vi "Initial_Plugin_Dynamixel.vi"() -> (5 "Plug in titles":string[](array[string]), 7 "Plug in values":string[](array[string]))   [LabVIEW 2022 SP3]
uses:
  Controls/Post_Process.ctl
  Controls/Setup.ctl
  Globals/Trav_pos_global.vi
  Globals/Meas_global.vi
  ADAM Serial/Instrument drivers/Dynamixel/Sub Vis/Dynamixel Global.vi
  <vilib>/ptbypt/NI_PtbyPt.lvlib
panel:
  out "On This Block":i32
  out "Amplitude":dbl
  out "Centre":dbl
  in  "Phase (Deg)":dbl
  in  "No of Cycles":dbl
  in  "Acceleration":dbl
  in  "Velocity":dbl
  in  "Min Peak":dbl
  in  "Max peak":dbl
  in  "Sinewave Freq (Hz)":dbl
  in  "Delay between Rendezvous and Acquisition starting (ms)":u32
  in  "Delay before each Traverse Move (ms)":u32=2000
  out "Position (Deg)":dbl
  out "Message":string
  out "Case Currently On":string
  # "The Vi\nEnFlo Software\\ADAM Serial\\Instrument drivers\\Dynamixel\\Dynamixel live Position Server.vi\nmust be running for this vi to work"
  # "Specific Arguments"
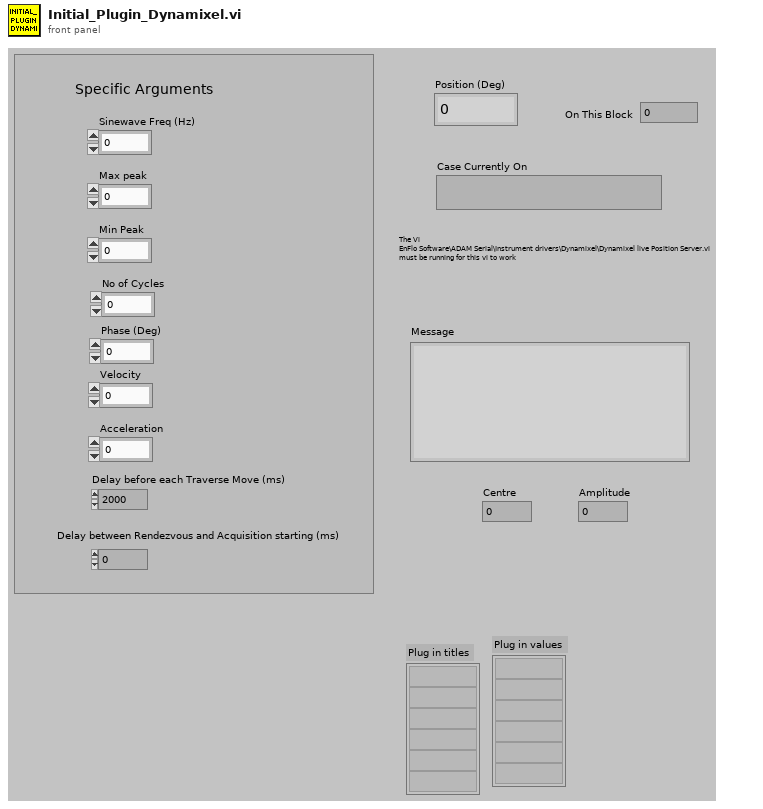
[diagram p1: front panel]
types:
  T1 = typedef "Traverse_cluster.ctl" = cluster{"Start X":sgl, "Start Y":sgl, "Start Z":sgl, "End X":sgl, "End Y":sgl, "End Z":sgl, "nPoints":i32, "Spacing":T2, "Filename":path, "Tunnel Speed":dbl, "Averaging time (mins)":dbl, "Extra Commands":string, "Carrier_1 Q (l/min)":dbl, "Carrier_2 Q (l/min)":dbl, "Trace Gas Concentration (%)":dbl, "Specific Arguments":string, "Comments":string, "Row No":i32, "Row Type Selector":T3, "EstCompl":string, "Row Duration (mins)":dbl, "nValidPoints":i32, "Meas Setup File":string}
  T2 = typedef "Spacing.ctl" = enum16{"Linear", "Log", "Gauss", "Specified", "N/A"}
  T3 = typedef "Multi_run_mode.ctl" = enum16{"Move Traverse Only", "Set Tunnel Speed Only", "Set Source Only", "Set Measurement Conditions", "Single Measurement", "Vertical Profile", "Lateral Profile", "Longitudinal Profile", "Multi-Axis Profile", "Explore Volume", "Auto Calibrate", "Meas Fast FID Bkgnd", "Check Beam Power", "Scanning Valve Measurement", "Run VI Named:", "Set ADAM Ch", "Wait (minutes)", "Send Message", "Synchronize With:", "Fall Back to this Row", "Turn Off Row Repeating", "Traverse 3D Volume", "Blank Row", "Jump to Fall Back Row"}
  T4 = typedef "Post_Process.ctl" = enum16{"Take New Data", "Post Process Raw Data File"}
  T5 = typedef "Setup.ctl" = enum16{"Run Program", "Show Setup", "Save Current Setup", "Setup Front Panel"}
  T6 = typedef "Rendezvous RefNum" = refnum<k1>
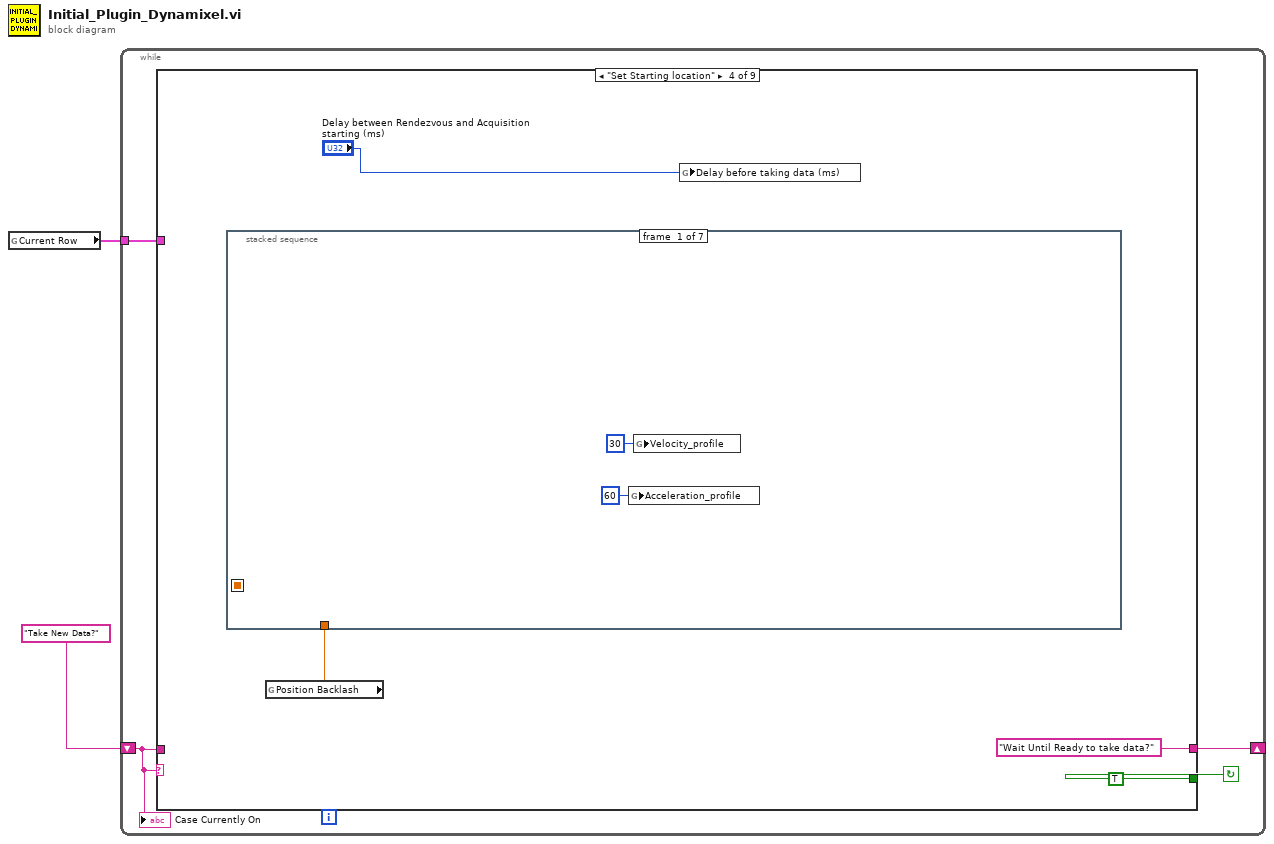
[diagram p0: block diagram]
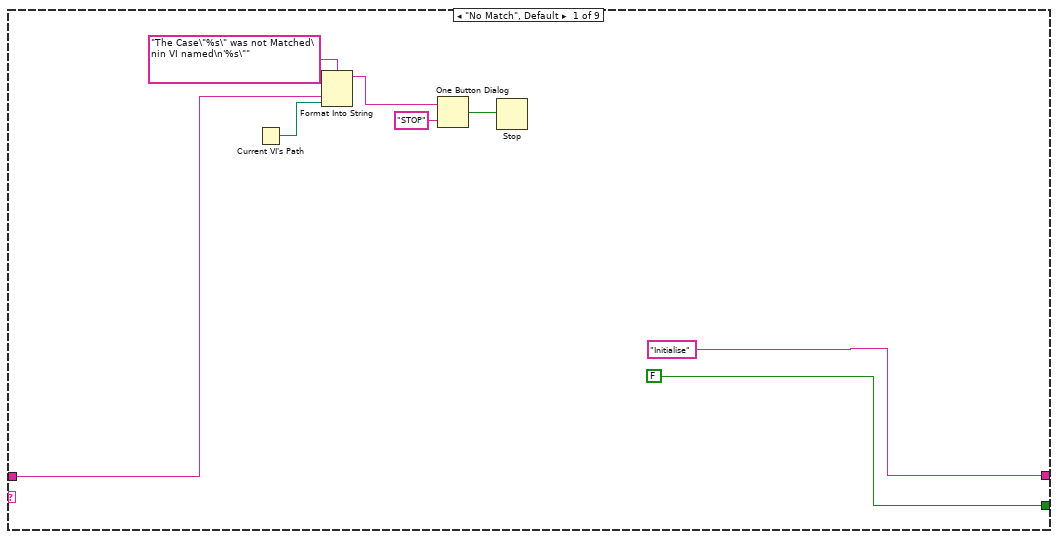
[diagram p2: hidden frame]
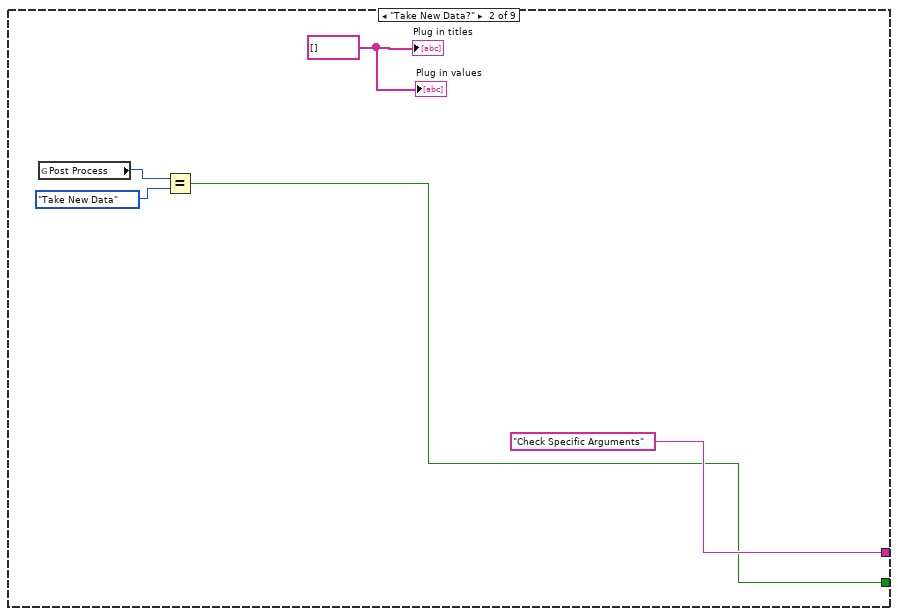
[diagram p3: hidden frame]
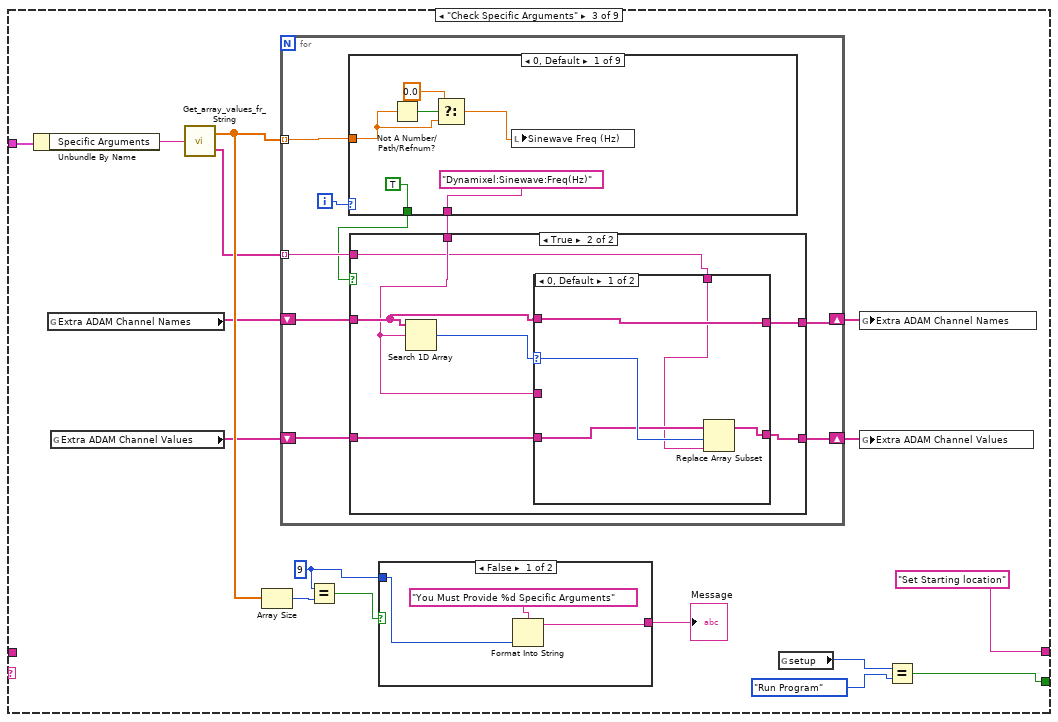
[diagram p4: hidden frame]
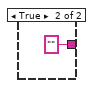
[diagram p5: hidden frame]
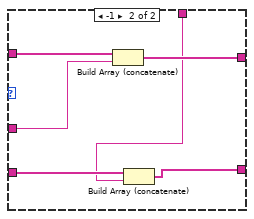
[diagram p7: hidden frame]
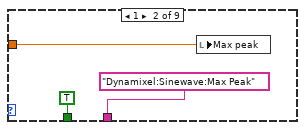
[diagram p8: hidden frame]
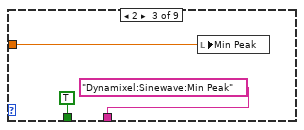
[diagram p9: hidden frame]
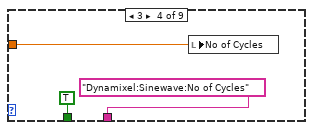
[diagram p10: hidden frame]
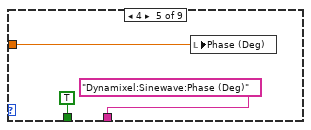
[diagram p11: hidden frame]
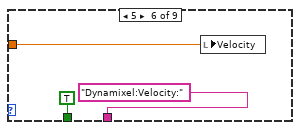
[diagram p12: hidden frame]
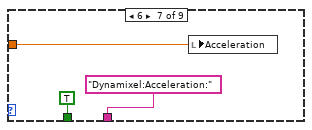
[diagram p13: hidden frame]
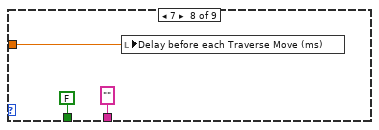
[diagram p14: hidden frame]
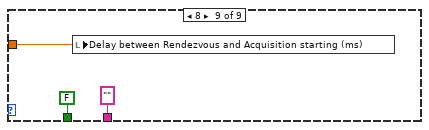
[diagram p15: hidden frame]
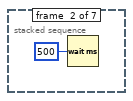
[diagram p16: hidden frame]
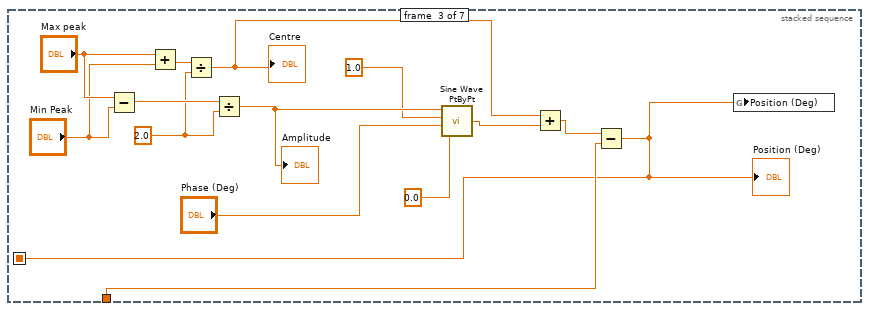
[diagram p17: hidden frame]
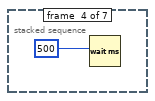
[diagram p18: hidden frame]
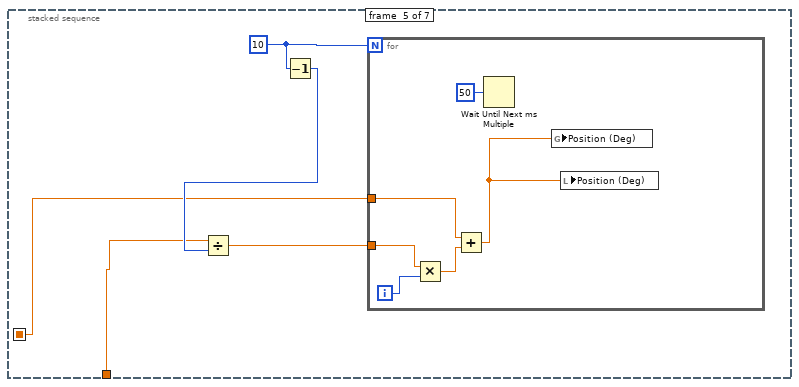
[diagram p19: hidden frame]
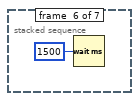
[diagram p20: hidden frame]
diagram:
  n1 = global read "Trav_pos_global.vi" "Current Row"() -> (w1:T1)
  n2 = while {
    shift-left: "Take New Data?" -> [w4]
    shift-right: [w5] -> _
    tunnel: w1 -> [w3]
    stop <- w6 continue-if-true
    n3 = case shown="\"Set Starting location\"" w4 {
      tunnel: [FALSE w15 w21 TRUE ("Command Found") TRUE ("Command Found") TRUE ("Command Found") TRUE ("Command Found") TRUE ("Command Found") FALSE ("Command Found")] -> w6
      tunnel: ["Initialise" "Check Specific Arguments" "Set Starting location" ("f") "Wait Until Ready to take data?" ("f") w137 "Move Servo Motor" "Another Block?" w180 "End" ("f")] -> w5
      tunnel: w4 -> [w9 _ _ _ _ _ _ _ _]
      tunnel: w3 -> [_ _ w34 _ _ _ _ _ _]
      frame "No Match", Default {
        n4 = Current VI's Path() -> (path=w8:path)
        n5 = Format Into String(format string="The Case\"%s\" was not Matched\nin VI named\n'%s\"" ("Format String"), w9, w8) -> (resulting string=w12:string)  [unwired: 2 in, 1 out]
        n6 = One Button Dialog(message=w12, button name ("OK")="STOP") -> (true=w10:bool)
        n7 = Stop(stop? (T)=w10) -> ()
      }
      frame "Take New Data?" {
        w16 = string[] [] ("Plug in titles")
        n8 = global read "Meas_global.vi" "Post Process"() -> (w18:T4)
        n9 = Equal?(x=w18, y=Post_Process."Take New Data" ("Post Process")) -> (x = y?=w15:bool)
        "Plug in titles" <- w16
        "Plug in values" <- w16
      }
      frame "Check Specific Arguments" {
        w20 = 9 ("x")
        n10 = Unbundle By Name(w34) -> ("Specific Arguments"=w35:string)
        n11 = global read "Meas_global.vi" "Extra ADAM Channel Names"() -> (w28:string[])
        n12 = global read "Meas_global.vi" "Extra ADAM Channel Values"() -> (w25:string[])
        n13 = call "Get_array_values_fr_String.vi"("String Value"=w35) -> ("Numeric Array"=w32:dbl[], "String array"=w24:string[])
        n14 = Array Size(array=w32) -> (size(s)=w31:i32)
        n15 = for {
          tunnel: w32 -> [w47] mode=indexing
          shift-right: [w45] -> w27
          shift-left: w28 -> [w46]
          shift-right: [w42] -> w26
          shift-left: w25 -> [w43]
          tunnel: w24 -> [w41] mode=indexing
          i -> [w48]
          n16 = case shown="0, Default" w48 {
            tunnel: w47 -> [w71 w77 w80 w83 w86 w87 w90 w95 w98]
            tunnel: ["Dynamixel:Sinewave:Freq(Hz)" "Dynamixel:Sinewave:Max Peak" "Dynamixel:Sinewave:Min Peak" "Dynamixel:Sinewave:No of Cycles" "Dynamixel:Sinewave:Phase (Deg)" "Dynamixel:Velocity:" "Dynamixel:Acceleration:" "" ""] -> w44
            tunnel: [TRUE TRUE TRUE TRUE TRUE TRUE TRUE FALSE FALSE] -> w40
            frame 0, Default {
              n17 = Not A Number/Path/Refnum?(number/path/refnum=w71) -> (NaN/Path/Refnum?=w72:bool)
              n18 = Select(t=0.0, s=w72, f=w71) -> (s? t:f=w70:dbl)
              n19 = local write "Sinewave Freq (Hz)"(w70) -> ()
            }
            frame 1 {
              n20 = local write "Max peak"(w77) -> ()
            }
            frame 2 {
              n21 = local write "Min Peak"(w80) -> ()
            }
            frame 3 {
              n22 = local write "No of Cycles"(w83) -> ()
            }
            frame 4 {
              n23 = local write "Phase (Deg)"(w86) -> ()
            }
            frame 5 {
              n24 = local write "Velocity"(w87) -> ()
            }
            frame 6 {
              n25 = local write "Acceleration"(w90) -> ()
            }
            frame 7 {
              n26 = local write "Delay before each Traverse Move (ms)"(w95) -> ()
            }
            frame 8 {
              n27 = local write "Delay between Rendezvous and Acquisition starting (ms)"(w98) -> ()
            }
          }
          n28 = case shown="True" w40 {
            tunnel: w46 -> [w50 w57]
            tunnel: [w50 w56] -> w45
            tunnel: w44 -> [_ w55]
            tunnel: w43 -> [w49 w53]
            tunnel: [w49 w52] -> w42
            tunnel: w41 -> [_ w51]
            frame False {
            }
            frame True {
              n29 = Search 1D Array(1D array=w57, element=w55) -> (index of element=w54:i32)  [unwired: 1 in]
              n30 = case shown="0, Default" w54 {
                selector: w54 -> [w61 _]
                tunnel: w57 -> [w62 w68]
                tunnel: w55 -> [_ w67]
                tunnel: [w62 w66] -> w56
                tunnel: w53 -> [w60 w65]
                tunnel: [w59 w64] -> w52
                tunnel: w51 -> [w58 w63]
                frame 0, Default {
                  n31 = Replace Array Subset(array=w60, new element=w58, index=w61) -> (w59:string[])
                }
                frame -1 {
                  n32 = Build Array (concatenate)(w68, w67) -> (w66:string[])
                  n33 = Build Array (concatenate)(w65, w63) -> (w64:string[])
                }
              }
            }
          }
        }
        n34 = Equal?(x=w20, y=w31) -> (x = y?=w30:bool)
        n35 = case shown="False" w30 {
          tunnel: [w36 ""] -> w29
          tunnel: w20 -> [w37 _]
          frame False {
            n36 = Format Into String(format string="You Must Provide %d Specific Arguments", w37) -> (resulting string=w36:string)  [unwired: 2 in, 1 out]
          }
          frame True {
          }
        }
        "Message" <- w29
        n37 = global read "Meas_global.vi" "setup"() -> (w23:T5)
        n38 = global write "Meas_global.vi" "Extra ADAM Channel Names"(w27) -> ()
        n39 = global write "Meas_global.vi" "Extra ADAM Channel Values"(w26) -> ()
        n40 = Equal?(x=w23, y=Setup."Run Program" ("setup")) -> (x = y?=w21:bool)
      }
      frame "Set Starting location" {
        n41 = global read "Dynamixel Global.vi" "Position Backlash"() -> (w99:dbl)
        n42 = stacked-sequence {
          seq-local: [_ _ w106 _ _ _ _] -> [_ _ _ _ w121 _ _]
          tunnel: w99 -> [_ _ w107 _ w122 _ _]
          frame #0 {
            n43 = global write "Dynamixel Global.vi" "Acceleration_profile"(u32 60 ("Acceleration_profile")) -> ()
            n44 = global write "Dynamixel Global.vi" "Velocity_profile"(u32 30 ("Velocity_profile")) -> ()
          }
          frame #1 {
            n45 = Wait (ms)(milliseconds to wait=u32 500) -> ()  [unwired: 1 out]
          }
          frame #2 {
            w115 = 2.0 ("y")
            n46 = Subtract(x="Max peak", y="Min Peak") -> (x-y=w119:dbl)
            n47 = Add(x="Max peak", y="Min Peak") -> (x+y=w116:dbl)
            n48 = Divide(x=w116, y=w115) -> (x/y=w109:dbl)
            "Centre" <- w109
            n49 = Divide(x=w119, y=w115) -> (x/y=w114:dbl)
            "Amplitude" <- w114
            n50 = call <vilib>:"Sine Wave PtByPt.vi"("time"=0.0, "phase"="Phase (Deg)", "frequency"=1.0, "amplitude"=w114) -> ("sine wave"=w110:dbl)
            n51 = Add(x=w109, y=w110) -> (x+y=w108:dbl)
            n52 = Subtract(x=w108, y=w107) -> (x-y=w106:dbl)
            "Position (Deg)" <- w106
            n53 = global write "Dynamixel Global.vi" "Position (Deg)"(w106) -> ()
          }
          frame #3 {
            n54 = Wait (ms)(milliseconds to wait=u32 500 ("millisecond timer value")) -> ()  [unwired: 1 out]
          }
          frame #4 {
            w124 = 10
            n55 = Decrement(x=w124) -> (x-1=w123:i32)
            n56 = Divide(x=w122, y=w123) -> (x/y=w125:dbl)
            n57 = for {
              N: w124 -> [_]
              tunnel: w125 -> [w130]
              tunnel: w121 -> [w128]
              i -> [w131]
              n58 = Multiply(x=w130, y=w131) -> (x*y=w129:dbl)
              n59 = Add(x=w128, y=w129) -> (x+y=w127:dbl)
              n60 = Wait Until Next ms Multiple(millisecond multiple=u32 50) -> ()  [unwired: 1 out]
              n61 = global write "Dynamixel Global.vi" "Position (Deg)"(w127) -> ()
              n62 = local write "Position (Deg)"(w127) -> ()
            }
          }
          frame #5 {
            n63 = Wait (ms)(milliseconds to wait=u32 1500) -> ()  [unwired: 1 out]
          }
          frame #6 {
            n64 = global write "Dynamixel Global.vi" "Velocity_profile"("Velocity") -> ()
            n65 = global write "Dynamixel Global.vi" "Acceleration_profile"("Acceleration") -> ()
          }
        }
        n66 = global write "Meas_global.vi" "Delay before taking data (ms)"("Delay between Rendezvous and Acquisition starting (ms)") -> ()
      }
      frame "Wait Until Ready to take data?" {
        n67 = global read "Meas_global.vi" "Acquisition Rendezvous"() -> (w139:T6)
        n68 = call <vilib>:"Wait at Rendezvous.vi"("ms timeout (-1)"=60000, "rendezvous"=w139) -> ("error out"=w138:errorcluster)  [unwired: 3 in, 2 out]
        n69 = Unbundle By Name(w138) -> ("status"=w136:bool)
        n70 = case shown="True" w136 {
          tunnel: ["Delay before moving Servo motor" "Wait Until Ready to take data?"] -> w137
          frame False {
          }
          frame True {
            # "This is to wait for the Acquisition Rendexvous to become live"
          }
        }
      }
      frame "Delay before moving Servo motor" {
        n71 = global read "Meas_global.vi" "Current Block No"() -> (→"On This Block":i32)
        n72 = Wait (ms)(milliseconds to wait="Delay before each Traverse Move (ms)") -> ()  [unwired: 1 out]
      }
      frame "Move Servo Motor" {
        n73 = local read "Phase (Deg)"() -> (w147:dbl)
        n74 = Divide(x="No of Cycles", y="Sinewave Freq (Hz)") -> (x/y=w151:dbl)
        n75 = local read "Amplitude"() -> (w149:dbl)
        n76 = local read "Centre"() -> (w148:dbl)
        n77 = Multiply(x=w151, y=1000.0) -> (x*y=w152:dbl)
        n78 = Equal To 0?(x="Sinewave Freq (Hz)") -> (x = 0?=w155:bool)
        n79 = case shown="True" w155 {
          tunnel: "Sinewave Freq (Hz)" -> [w163 _]
          tunnel: w149 -> [w162 _]
          tunnel: w148 -> [w161 w179]
          tunnel: w152 -> [w160 _]
          tunnel: w147 -> [w158 _]
          frame False {
            n80 = To Long Integer(number=w160) -> (32bit integer=w159:i32)
            n81 = Tick Count (ms)() -> (millisecond timer value=w164:u32)
            n82 = while {
              tunnel: w164 -> [w177]
              tunnel: w163 -> [w173]
              tunnel: w162 -> [w172]
              tunnel: w161 -> [w170]
              tunnel: w159 -> [w168]
              tunnel: w158 -> [w165]
              stop <- w167 continue-if-true
              n83 = Tick Count (ms)() -> (millisecond timer value=w178:u32)
              n84 = Subtract(x=w178, y=w177) -> (x-y=w169:u32)
              n85 = Less?(x=w169, y=w168) -> (x < y?=w167:bool)
              n86 = Divide(x=w169, y=u32 1000) -> (x/y=w175:dbl)
              n87 = Wait Until Next ms Multiple(millisecond multiple=u32 3) -> ()  [unwired: 1 out]
              n88 = call <vilib>:"Sine Wave PtByPt.vi"("time"=w175, "phase"=w165, "frequency"=w173, "amplitude"=w172) -> ("sine wave"=w171:dbl)
              n89 = Add(x=w170, y=w171) -> (x+y=w166:dbl)
              n90 = local write "Position (Deg)"(w166) -> ()
              n91 = global write "Dynamixel Global.vi" "Position (Deg)"(w166) -> ()
            }
          }
          frame True {
            n92 = global write "Dynamixel Global.vi" "Position (Deg)"(w179) -> ()
            n93 = local write "Position (Deg)"(w179) -> ()
          }
        }
      }
      frame "Another Block?" {
        n94 = global read "Meas_global.vi" "Current Block No"() -> (w184:i32)
        n95 = global read "Meas_global.vi" "Requested No of blocks"() -> (w188:i32)
        n96 = local read "On This Block"() -> (w182:i32)
        n97 = Greater Or Equal?(x=w182, y=w188) -> (x >= y?=w187:bool)
        n98 = Equal?(x=w184, y=w182) -> (x = y?=w183:bool)
        n99 = case shown="False" w183 {
          tunnel: ["Set Starting location" ("f") "Another Block?"] -> w181
          frame False {
          }
          frame True {
            n100 = Wait (ms)(milliseconds to wait=u32 10) -> ()  [unwired: 1 out]
          }
        }
        n101 = Select(t="End", s=w187, f=w181) -> (s? t:f=w180:string)
      }
      frame "End" {
      }
    }
    "Case Currently On" <- w4
  }
